vi "标签流水号.vi"(8 "左真右假":bool, 11 "选择的型号":string="config\\BarcodeTemplate") -> (3 "数值":i32)   [LabVIEW 2018]
uses:
  <userlib>/_OpenG.lib/file/file.llb/File Exists - Scalar__ogtk.vi
  <vilib>/Utility/file.llb/Read Delimited Spreadsheet (string).vi
  <vilib>/Utility/file.llb/Write Delimited Spreadsheet (string).vi
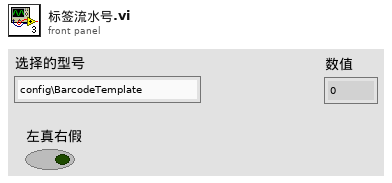
[diagram p1: front panel]
types:
  T1 = enum16{"open", "replace", "create", "open or create", "replace or create", "replace or create with confirmation"}
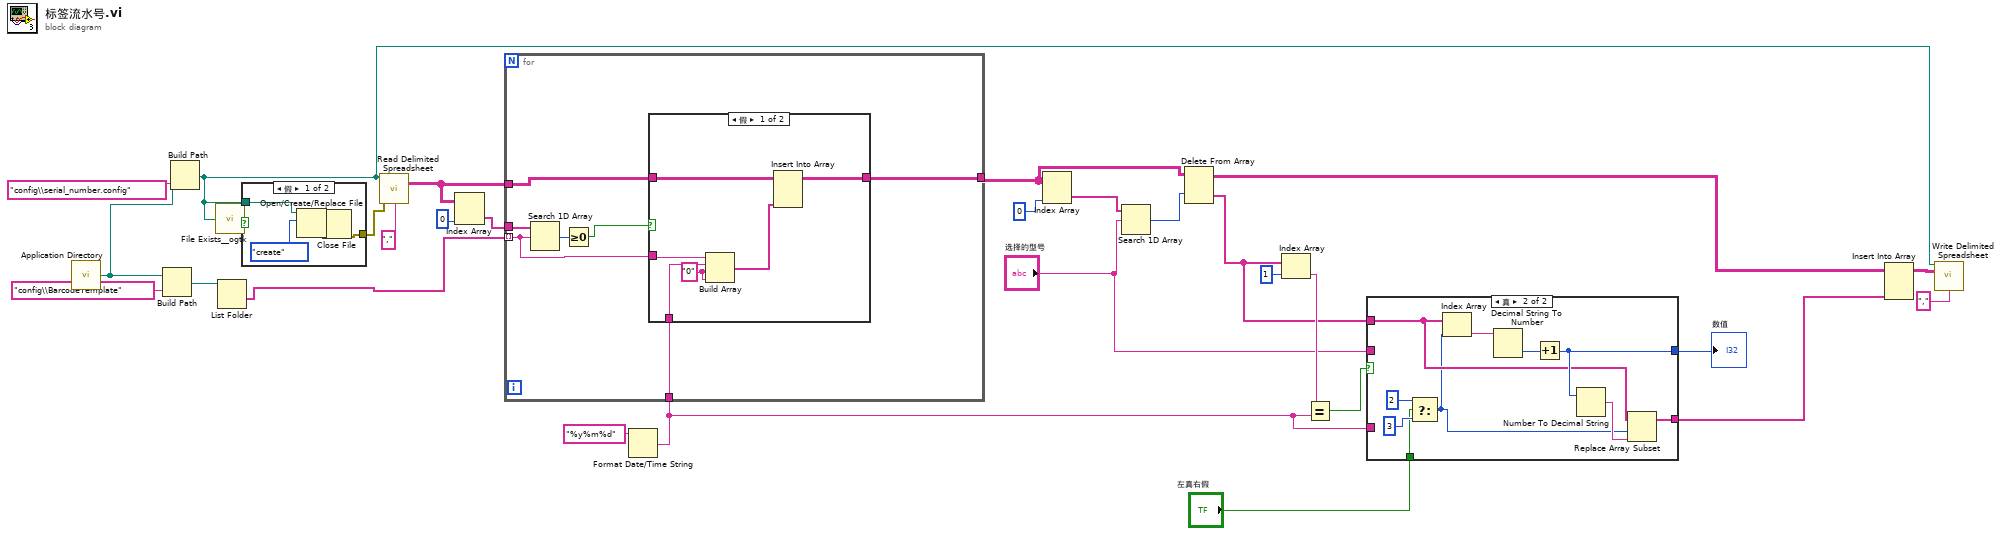
[diagram p0: block diagram]
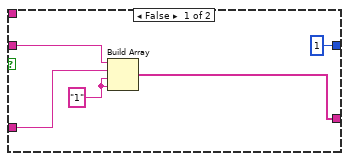
[diagram p2: hidden frame]
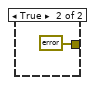
[diagram p3: hidden frame]
diagram:
  n1 = call <vilib>:"Application Directory.vi"() -> ("Application Directory"=w25:path)
  n2 = Build Path(base path=w25, name or relative path="config\\BarcodeTemplate" ("名称或相对路径")) -> (appended path=w26:path)
  n3 = Build Path(base path=w25, name or relative path="config\\serial_number.config" ("名称或相对路径")) -> (appended path=w1:path)
  n4 = call-poly <userlib>:"File Exists__ogtk.vi"("file path"=w1) -> ("exists"=w17:bool)  [unwired: 6 in, 1 out]
  n5 = List Folder(path=w26) -> (folder names=w15:string[])  [unwired: 3 in, 3 out]
  n6 = case shown="假" w17 {
    tunnel: w1 -> [w34 _]
    tunnel: [w30 errorcluster {"status"=FALSE, "code"=0, "source"=""} ("error out")] -> w16
    frame False {
      n7 = Open/Create/Replace File(file path (use dialog)=w34, operation (0:open)=T1."create" ("操作(0:open)")) -> (refnum out=w32:refnum<file>, error out=w31:errorcluster)  [unwired: 4 in, 1 out]
      n8 = Close File(refnum=w32, error in=w31) -> (error out=w30:errorcluster)  [unwired: 1 out]
    }
    frame True {
    }
  }
  n9 = call-poly <vilib>:"Read Delimited Spreadsheet.vi"("file path (dialog if empty)"=w1, "error in (no error)"=w16, "delimiter (\\t)"="," ("delimiter (\\t)")) -> ("all rows"=w22:string[][])  [unwired: 7 in, 5 out]
  n10 = Index Array(array=w22, index (col)=0 ("禁用的索引 (列)")) -> (element=w23:string[])  [unwired: 1 in]
  n11 = Format Date/Time String(time format string (%c)="%y%m%d" ("时间格式字符串(%c)")) -> (date/time string=w5:string)  [unwired: 2 in]
  n12 = for {
    tunnel: w23 -> [w40]
    tunnel: w15 -> [w38] mode=indexing
    tunnel: w22 -> [w39]
    tunnel: w5 -> [w37]
    tunnel: [w36] -> w19
    n13 = Search 1D Array(1D array=w40, element=w38) -> (index of element=w42:i32)  [unwired: 1 in]
    n14 = Greater Or Equal To 0?(x=w42) -> (x >= 0?=w41:bool)
    n15 = case shown="假" w41 {
      tunnel: w39 -> [w48 w49]
      tunnel: w38 -> [w47 _]
      tunnel: w37 -> [w46 _]
      tunnel: [w43 w49] -> w36
      frame False {
        w45 = "0" ("元素")
        n16 = Build Array(w47, w46, w45, w45) -> (w44:string[])
        n17 = Insert Into Array(array=w48, new element=w44) -> (w43:string[][])  [unwired: 2 in]
      }
      frame True {
      }
    }
  }
  n18 = Index Array(array=w19, index (col)=0 ("禁用的索引 (列)")) -> (element=w20:string[])  [unwired: 1 in]
  n19 = Search 1D Array(1D array=w20, element="选择的型号") -> (index of element=w10:i32)  [unwired: 1 in]
  n20 = Delete From Array(array=w19, index (row)=w10) -> (deleted portion=w9:string[], array with subset deleted=w7:string[][])  [unwired: 2 in]
  n21 = Index Array(array=w9, index=1 ("索引")) -> (element=w13:string)
  n22 = Equal?(x=w13, y=w5) -> (x = y?=w12:bool)
  n23 = case shown="真" w12 {
    tunnel: w9 -> [_ w58]
    tunnel: "左真右假" -> [_ w63]
    tunnel: [1 w59] -> w8
    tunnel: [w51 w55] -> w6
    tunnel: w5 -> [w53 _]
    tunnel: "选择的型号" -> [w54 _]
    frame False {
      w52 = "1" ("元素")
      n24 = Build Array(w54, w53, w52, w52) -> (w51:string[])
    }
    frame True {
      n25 = Select(t=2 ("禁用的索引 (列)"), s=w63, f=3 ("禁用的索引 (列)")) -> (s? t:f=w56:i32)
      n26 = Index Array(array=w58, index=w56) -> (element=w61:string)
      n27 = Decimal String To Number(string=w61) -> (number=w60:i32)  [unwired: 2 in, 1 out]
      n28 = Increment(x=w60) -> (x+1=w59:i32)
      n29 = Number To Decimal String(number=w59) -> (decimal integer string=w57:string)  [unwired: 1 in]
      n30 = Replace Array Subset(array=w58, new element=w57, index=w56) -> (w55:string[])
    }
  }
  "数值" <- w8
  n31 = Insert Into Array(array=w7, new element=w6) -> (w3:string[][])  [unwired: 2 in]
  n32 = call-poly <vilib>:"Write Delimited Spreadsheet.vi"("file path (dialog if empty)"=w1, "2D data"=w3, "delimiter (\\t)"="," ("delimiter (\\t)")) -> ()  [unwired: 11 in, 2 out]
